vi "RemoteDCPowerSession_CallCloseMeasurementLinkSessionWithDetachBehavior_RemoteSessionDetached.vi"(8 "error in":errorcluster) -> (0 "error out":errorcluster, 2 "result":string, 3 "pass":bool)   [LabVIEW 2020, in "MeasurementServerTests.lvlib"]
uses:
  MeasurementServerTests.lvlib
  Runtime/MeasurementLink niDCPower/Instrument/Instrument.lvclass
  Runtime/MeasurementLink Instrument/IInstrument/Close Session Behavior.ctl
  Runtime/MeasurementLink Instrument/IInstrument/IInstrument.lvclass
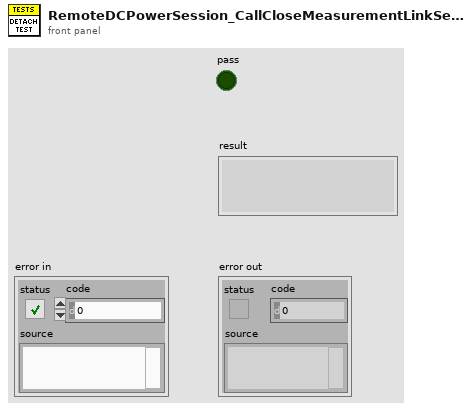
[diagram p1: front panel]
types:
  T1 = typedef "MeasurementLink Instrument.lvlib/IInstrument.lvclass/Remote Connection Options.ctl" = cluster{"session name":string, "address":string, "port":u32}
  T2 = typedef "MeasurementLink Instrument.lvlib/IInstrument.lvclass/Close Session Behavior.ctl" = enum16{"Close Session", "Detach Session"}
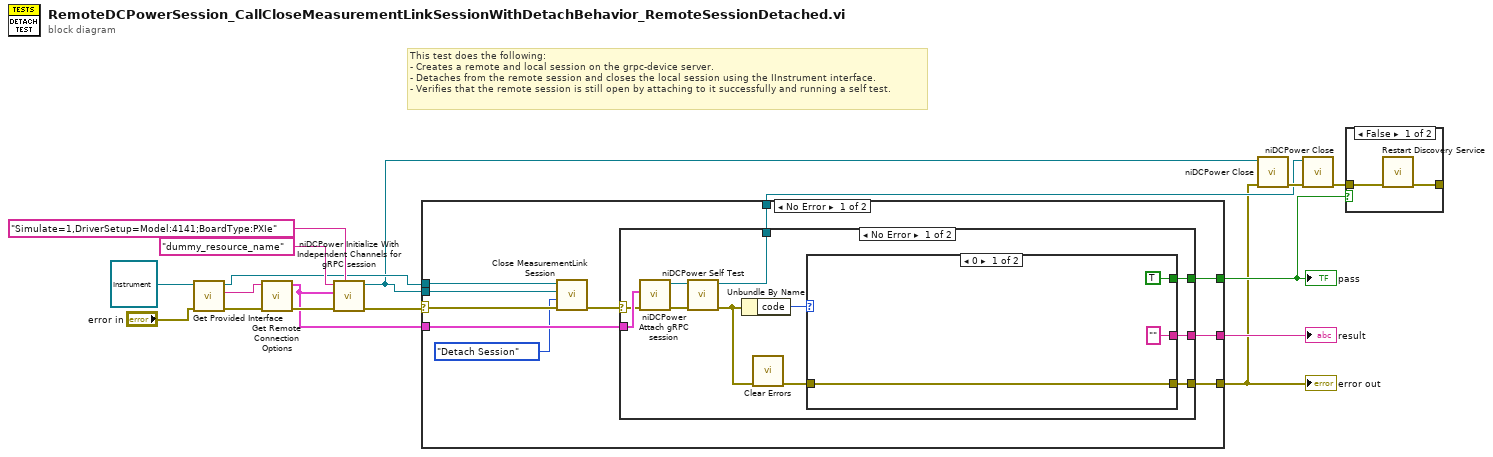
[diagram p0: block diagram]
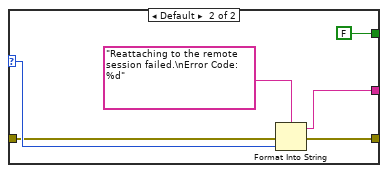
[diagram p3: hidden frame]
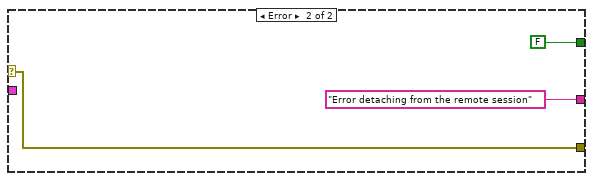
[diagram p4: hidden frame]
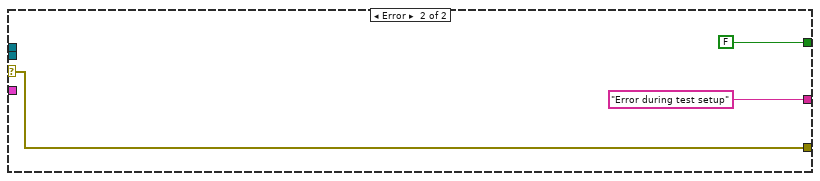
[diagram p5: hidden frame]
diagram:
  # "This test does the following:\n- Creates a remote and local session on the grpc-device server.\n- Detaches from the remote session and closes the local session using the IInstrument interface.\n- Verifies that the remote session is still open by attaching to it successfully and running a self test."
  n1 = call-dynamic "Get Provided Interface.vi"("error in"="error in", "instrument in"=refnum<class "Instrument.lvclass"> refnum ("MeasurementLink niDCPower.lvlib:Instrument.lvclass")) -> ("error out"=w14:errorcluster, "provided interface"=w13:string, "instrument out"=w9:refnum<class "Instrument.lvclass">)  [unwired: 7 in]
  n2 = call "Get Remote Connection Options.vi"("error in"=w14, "provided interface"=w13) -> ("error out"=w16:errorcluster, "remote connection options"=w8:T1)  [unwired: 8 in]
  n3 = call <instrlib>:"niDCPower Initialize With Independent Channels for gRPC session.vi"("option string"="Simulate=1,DriverSetup=Model:4141;BoardType:PXIe", "error in (no error)"=w16, "gRPC options"=w8, "resource name"="dummy_resource_name") -> ("error out"=w10:errorcluster, "instrument handle out"=w3:refnum<k15>)  [unwired: 6 in]
  n4 = case shown="No Error" w10 {
    selector: w10 -> [w27 w52]
    tunnel: w9 -> [w26 _]
    tunnel: w3 -> [w25 _]
    tunnel: w8 -> [w24 _]
    tunnel: [w22 w52] -> w1
    tunnel: [w21 FALSE] -> w4
    tunnel: [w20 "Error during test setup" ("f")] -> w7
    tunnel: [w18 _] -> w2
    frame No Error {
      n5 = call-dynamic "Close MeasurementLink Session.vi"("error in"=w27, "close session behavior"=Close_Session_Behavior."Detach Session", "session in"=w25, "instrument in"=w26) -> ("error out"=w23:errorcluster)  [unwired: 7 in]
      n6 = case shown="No Error" w23 {
        selector: w23 -> [w37 w48]
        tunnel: w24 -> [w38 _]
        tunnel: [w33 w48] -> w22
        tunnel: [w36 FALSE] -> w21
        tunnel: [w32 "Error detaching from the remote session" ("f")] -> w20
        tunnel: [w29 _] -> w18
        frame No Error {
          n7 = call <instrlib>:"niDCPower Attach gRPC session.vi"("error in (no error)"=w37, "gRPC options"=w38) -> ("error out"=w30:errorcluster, "instrument handle out"=w31:refnum<k15>)  [unwired: 8 in]
          n8 = call <instrlib>:"niDCPower Self Test.vi"("error in (no error)"=w30, "instrument handle"=w31) -> ("error out"=w28:errorcluster, "instrument handle out"=w29:refnum<k15>)  [unwired: 6 in, 2 out]
          n9 = Unbundle By Name(w28) -> ("code"=w35:i32)
          n10 = call <vilib>:"Clear Errors.vi"("error in (no error)"=w28) -> ("error out"=w34:errorcluster)  [unwired: 5 in, 1 out]
          n11 = case shown="0" w35 {
            selector: w35 -> [_ w46]
            tunnel: ["" ("f") w45] -> w32
            tunnel: [TRUE FALSE] -> w36
            tunnel: w34 -> [w40 w43]
            tunnel: [w40 w42] -> w33
            frame 0 {
            }
            frame Default {
              n12 = Format Into String(format string="Reattaching to the remote session failed.\nError Code: %d" ("f"), error in=w43, w46) -> (resulting string=w45:string, error out=w42:errorcluster)  [unwired: 1 in]
            }
          }
        }
        frame Error {
        }
      }
    }
    frame Error {
    }
  }
  "error out" <- w1
  "pass" <- w4
  "result" <- w7
  n13 = call <instrlib>:"niDCPower Close.vi"("error in (no error)"=w1, "instrument handle"=w3) -> ("error out"=w6:errorcluster)  [unwired: 9 in]
  n14 = call <instrlib>:"niDCPower Close.vi"("error in (no error)"=w6, "instrument handle"=w2) -> ("error out"=w5:errorcluster)  [unwired: 9 in]
  n15 = case shown="False" w4 {
    tunnel: [w55 _] -> _
    tunnel: w5 -> [w54 _]
    frame False {
      n16 = call "Restart Discovery Service.vi"("error in"=w54) -> ("error out"=w55:errorcluster)  [unwired: 10 in]
    }
    frame True {
    }
  }
